vi "DestroySelfReference.vi"(8 "error in (no error)":errorcluster, 11 "SMO.Example":refnum<class "SMO.TopLevel.lvclass">) -> (0 "error out":errorcluster, 3 "SMO.Example out":refnum<class "SMO.TopLevel.lvclass">)   [LabVIEW 2013, in "SMO.TopLevel.lvclass"]
uses:
  SMO.TopLevel.lvclass
  src/SMO/SMO.lvclass
  SMO.TopLevel.lvclass/SMO.TopLevel.ctl
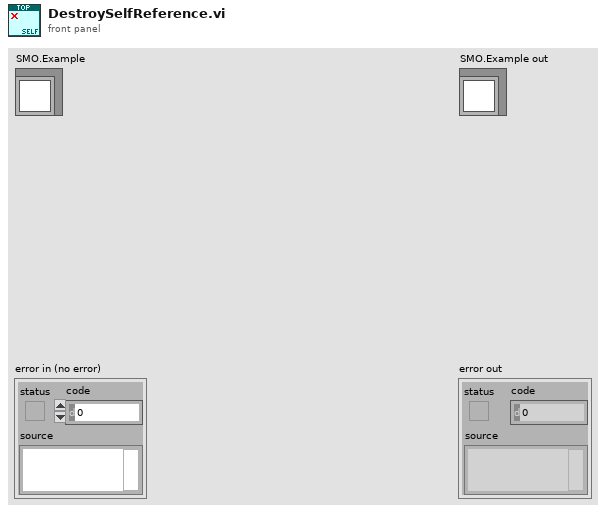
[diagram p1: front panel]
types:
  T1 = typedef "SMO.TopLevel.lvclass/PrivateData--Ref.ctl" = refnum<data-value>
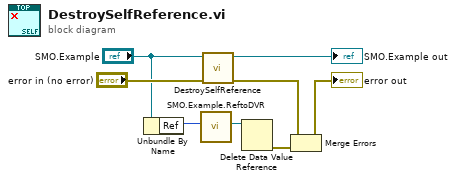
[diagram p0: block diagram]
diagram:
  n1 = Unbundle By Name("SMO.Example") -> ("Ref"=w2:u32)
  n2 = call "SMO.Example.ReftoDVR.vi"("Ref"=w2) -> ("Ref"=w1:T1)  [unwired: 10 in]
  n3 = call-parent "DestroySelfReference.vi"("error in (no error)"="error in (no error)", "SMO"="SMO.Example") -> ("error out"=w5:errorcluster, "SMO out"=→"SMO.Example out":refnum<class "SMO.TopLevel.lvclass">)  [unwired: 8 in]
  n4 = Delete Data Value Reference(data value reference=w1) -> (error out=w3:errorcluster)  [unwired: 1 in, 1 out]
  n5 = Merge Errors(w5, w3) -> (→"error out":errorcluster)
